vi "畫橢圓.vi"(8 "error in (no error)":errorcluster, 9 "Color":u32(colorbox)=16711680, 10 "Ellipse":T2 {"Minor Axis"."Point 2"."Y" format="%.2f"; "Minor Axis"."Point 2"."X" format="%.2f"; "Minor Axis"."Point 1"."Y" format="%.2f"; "Minor Axis"."Point 1"."X" format="%.2f"; "Major Axis"."Point 2"."Y" format="%.2f"; "Major Axis"."Point 2"."X" format="%.2f"; "Major Axis"."Point 1"."Y" format="%.2f"; "Major Axis"."Point 1"."X" format="%.2f"; "Center"."Y" format="%.2f"; "Center"."X" format="%.2f"}, 11 "Image In":T1) -> (0 "error out":errorcluster, 3 "Image":T1(plugin-control))   [LabVIEW 2015]
uses:
  <vilib>/vision/Image Controls.llb/IMAQ Image.ctl
panel:
  out "error out 2":errorcluster
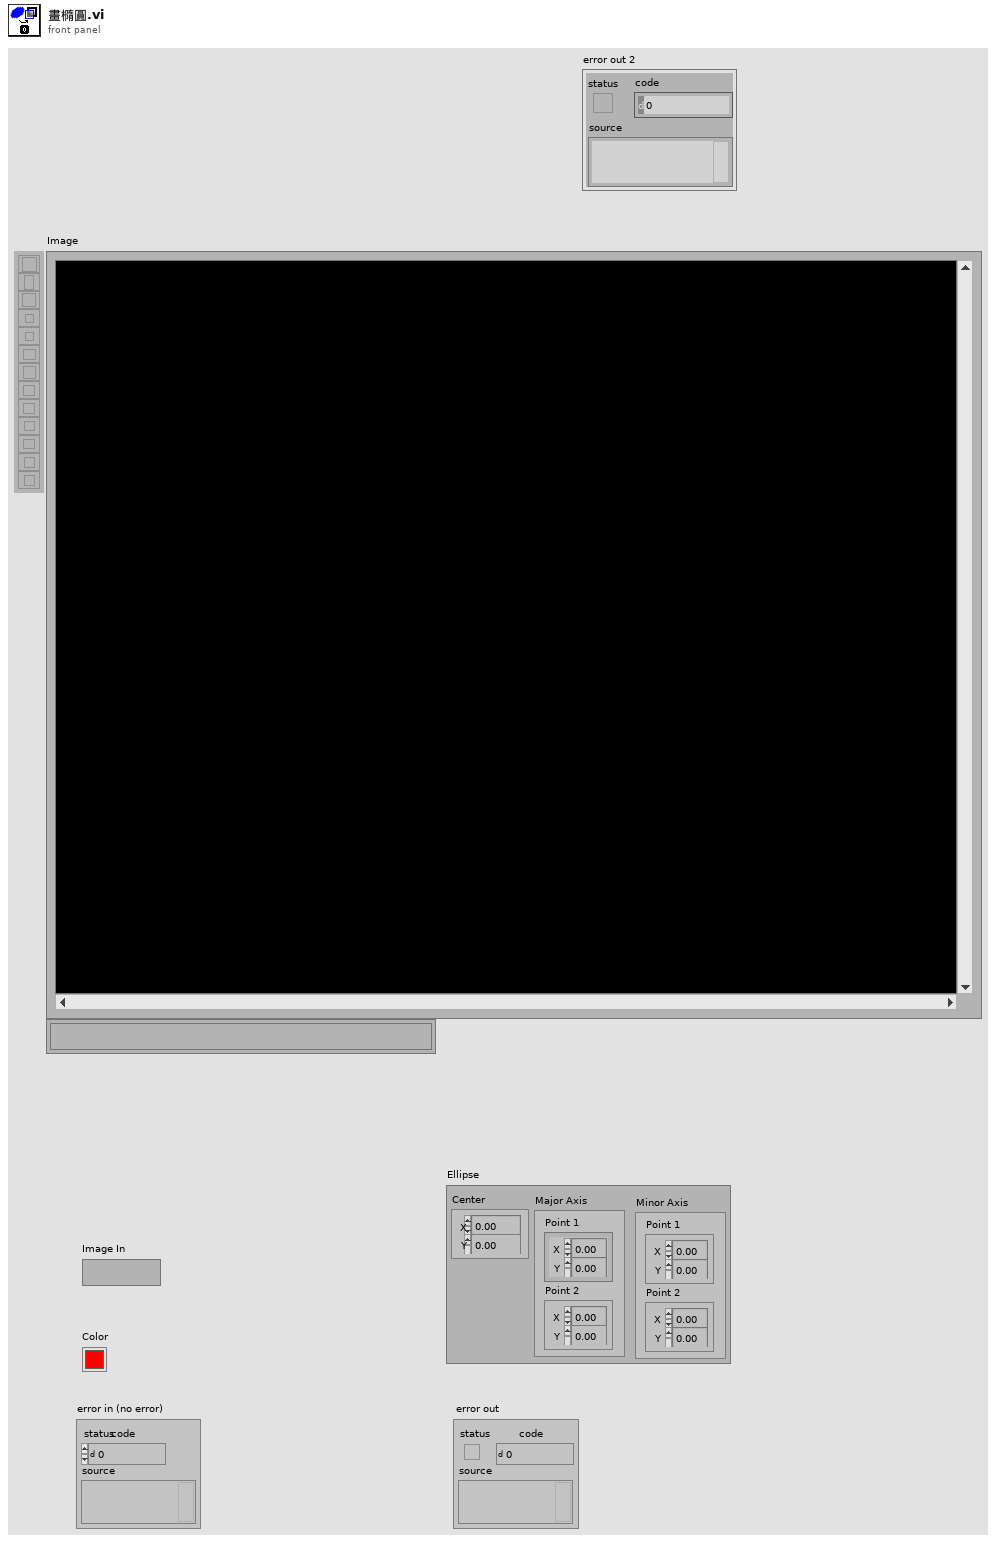
[diagram p1: front panel]
types:
  T1 = typedef "IMAQ Image.ctl" = refnum<image>
  T2 = cluster{"Center":cluster{"X":sgl, "Y":sgl}, "Major Axis":cluster{"Point 1":cluster{"X":sgl, "Y":sgl}, "Point 2":cluster{"X":sgl, "Y":sgl}}, "Minor Axis":cluster{"Point 1":cluster{"X":sgl, "Y":sgl}, "Point 2":cluster{"X":sgl, "Y":sgl}}}
  T3 = cluster{"Point 1":cluster{"X":sgl, "Y":sgl}, "Point 2":cluster{"X":sgl, "Y":sgl}}
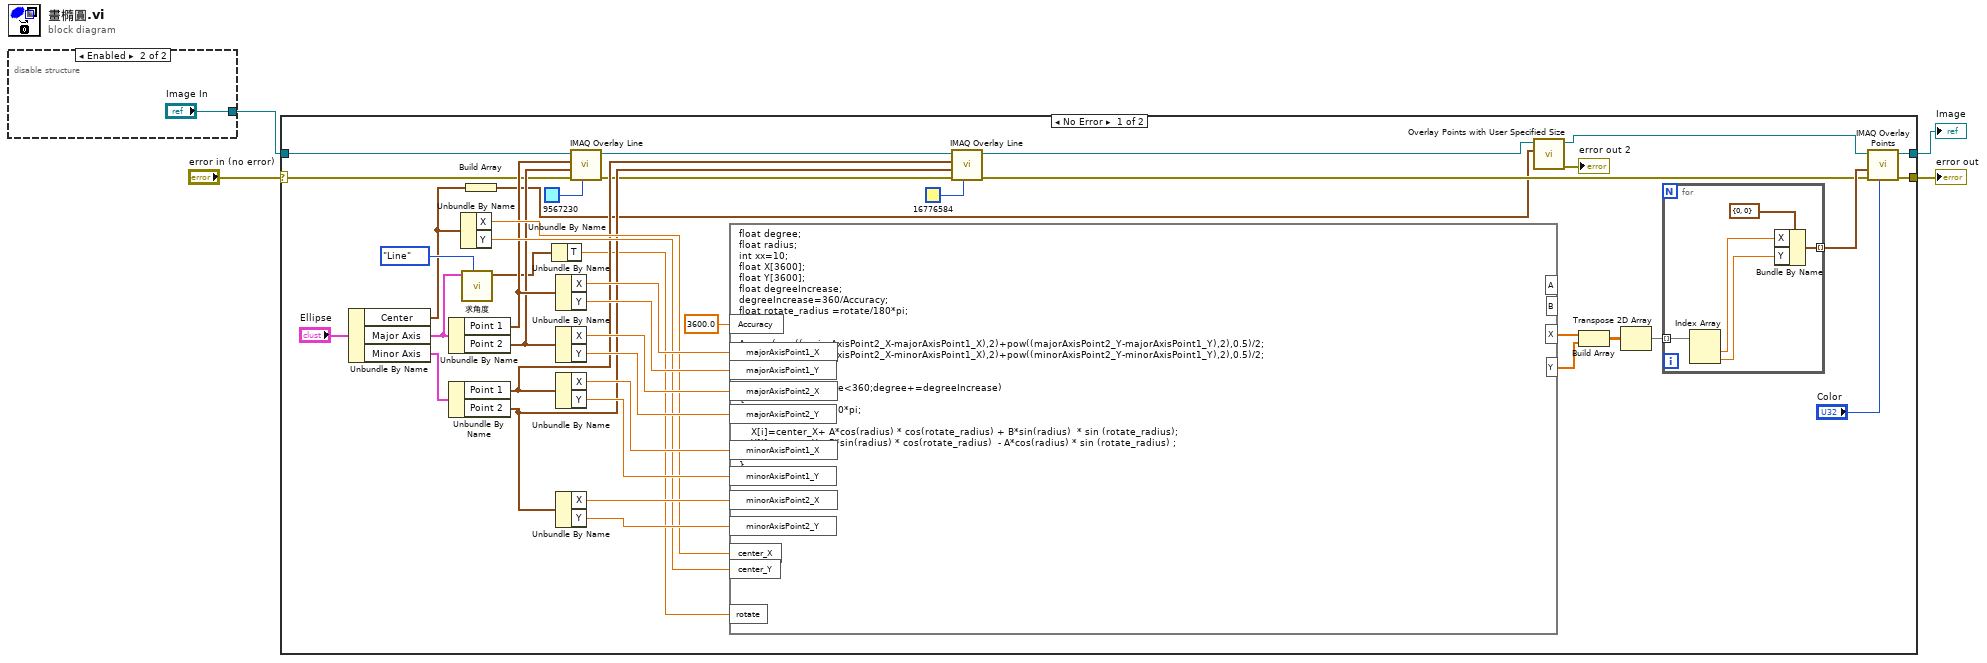
[diagram p0: block diagram]
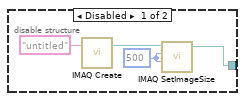
[diagram p3: hidden frame]
diagram:
  n1 = disable-structure shown="Enabled" {
    disable-tunnel: [w5 "Image In"] -> w3
    frame Disabled {
      w6 = 500 ("X Resolution")
      n2 = call "IMAQ Create"("Image Name"="untitled") -> ("New Image"=w7:T1)  [unwired: 4 in, 1 out]
      n3 = call "IMAQ SetImageSize"("Y Resolution"=w6, "X Resolution"=w6, "Image"=w7) -> ("Image Out"=w5:T1)  [unwired: 2 in, 1 out]
    }
    frame Enabled {
    }
  }
  n4 = case shown="No Error" "error in (no error)" {
    selector: "error in (no error)" -> [w10 w56]
    tunnel: [w38 w57] -> w4
    tunnel: w3 -> [w35 w57]
    tunnel: [w23 w56] -> w2
    frame No Error {
      n5 = Unbundle By Name("Ellipse") -> ("Center"=w15:cluster{"X":sgl, "Y":sgl}, "Major Axis"=w26:T3, "Minor Axis"=w46:T3)
      n6 = Unbundle By Name(w26) -> ("Point 1"=w34:cluster{"X":sgl, "Y":sgl}, "Point 2"=w31:cluster{"X":sgl, "Y":sgl})
      n7 = Unbundle By Name(w46) -> ("Point 1"=w30:cluster{"X":sgl, "Y":sgl}, "Point 2"=w29:cluster{"X":sgl, "Y":sgl})
      n8 = Unbundle By Name(w15) -> ("X"=w41:sgl, "Y"=w40:sgl)
      n9 = call "求角度.vi"("Line form"=enum16{"Line", "Two Point"}."Line", "Line"=w26) -> ("Line Data"=w19:cluster{"X":sgl, "Y":sgl, "T":sgl})  [unwired: 9 in]
      n10 = Build Array(w15) -> (w14:cluster{"X":sgl, "Y":sgl}[])
      n11 = Unbundle By Name(w19) -> ("T"=w18:sgl)
      n12 = Unbundle By Name(w34) -> ("X"=w50:sgl, "Y"=w49:sgl)
      n13 = Unbundle By Name(w31) -> ("X"=w48:sgl, "Y"=w47:sgl)
      n14 = Unbundle By Name(w30) -> ("X"=w45:sgl, "Y"=w44:sgl)
      n15 = Unbundle By Name(w29) -> ("X"=w43:sgl, "Y"=w42:sgl)
      n16 = call "IMAQ Overlay Line"("Color"=u32 9567230, "error in (no error)"=w10, "End Point"=w31, "Start Point"=w34, "Image"=w35) -> ("error out"=w22:errorcluster, "Image Out"=w36:T1)  [unwired: 5 in]
      n17 = formula code="float degree;\nfloat radius;\nint xx=10;\nfloat X[3600];\nfloat Y[3600];\nfloat degreeIncrease;\ndegreeIncrease=360/Accuracy;\nfloat rotate_radius =rotate/180*pi;\nint i=0;\n\nA=pow(pow((majorAxisPoint2_X-majorAxisPoint1_X),2)+pow((majorAxisPoint2_Y-majorAxisPoint1_Y),2),0.5)/2;\nB=pow(pow((minorAxisPoint2_X-minorAxisPoint1_X),2)+pow((minorAxisPoint2_Y-minorAxisPoint1_Y),2),0.5)/2;\n\n\nfor (degree=0;degree<360;degree+=degreeIncrease)\n{\n    radius=degree/180*pi;\n\n    X[i]=center_X+ A*cos(radius) * cos(rotate_radius) + B*sin(radius)  * sin (rotate_radius);\n    Y[i]=center_Y+ B*sin(radius) * cos(rotate_radius)  - A*cos(radius) * sin (rotate_radius) ;\n    i++;\n}"("majorAxisPoint1_X"=w50, "majorAxisPoint1_Y"=w49, "majorAxisPoint2_X"=w48, "majorAxisPoint2_Y"=w47, "minorAxisPoint1_X"=w45, "minorAxisPoint1_Y"=w44, "minorAxisPoint2_X"=w43, "minorAxisPoint2_Y"=w42, "center_X"=w41, "center_Y"=w40, "rotate"=w18, "Accuracy"=3600.0 ("input variable")) -> ("X"=w25:dbl[], "Y"=w24:dbl[])  [unwired: 2 out]
      n18 = call "IMAQ Overlay Line"("Color"=u32 16776584, "error in (no error)"=w22, "End Point"=w29, "Start Point"=w30, "Image"=w36) -> ("error out"=w21:errorcluster, "Image Out"=w17:T1)  [unwired: 5 in]
      n19 = call "Overlay Points with User Specified Size.vi"("Points"=w14, "Image In"=w17) -> ("error out"=→"error out 2":errorcluster, "Image Out"=w16:T1)  [unwired: 8 in]
      n20 = Build Array(w25, w24) -> (w39:dbl[][])
      n21 = Transpose 2D Array(2D array=w39) -> (transposed array=w12:dbl[][])
      n22 = for {
        tunnel: w12 -> [w55] mode=indexing
        tunnel: [w54] -> w37 mode=indexing
        n23 = Index Array(array=w55) -> (element #1=w52:dbl, element #2=w51:dbl)  [unwired: 2 in]
        n24 = Bundle By Name(cluster=cluster{"X":i32, "Y":i32} {"X"=0, "Y"=0}, "X"=w52, "Y"=w51) -> (w54:cluster{"X":i32, "Y":i32})
      }
      n25 = call "IMAQ Overlay Points"("Color"="Color", "error in (no error)"=w21, "Array of Points"=w37, "Image"=w16) -> ("error out"=w23:errorcluster, "Image Out"=w38:T1)  [unwired: 6 in]
    }
    frame Error {
    }
  }
  "Image" <- w4
  "error out" <- w2
